vi "EXTI_IO_ISR.vi"(11 "Interrupt_Flag":T1) -> ()   [LabVIEW 2011]
uses:
  D:/National Instruments/LabVIEW 2011/Targets/Keil/Embedded/RealView/Generic/My_ARM_Starter_Board/STM32_DriverVI_Interface/Interrupt/Interrupt_ISR.ctl
  <vilib>/eio/EIO_TerminalDirection.ctl
  <vilib>/STM32_DriverVI_Interface_F4/Interrupt/Interrupt_Flag_F4.ctl
  <vilib>/STM32_DriverVI_Interface_F4/GPIO_EIO/GPI_EIO_Inner_F4.vi
  <vilib>/STM32_DriverVI_Interface_F4/GPIO_EIO/GPO_EIO_Inner_F4.vi
  <vilib>/eio/EIONode/EIONode.xnode
panel:
  # "说明：\n这是一个标准的中断模板 VI，用户可以直接使用,\n在相应的Case语句里面实现相应的中断服务程序即可！\n\n双击打开这个VI之后，另存为副本，名称不变，将其保存\n并添加到自己的项目浏览器中，然后在程序生成规范中进行\n属性设置！"
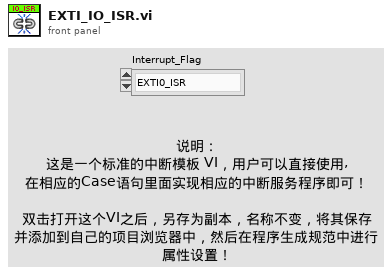
[diagram p1: front panel]
types:
  T1 = typedef "Interrupt_ISR.ctl" = enum8{"EXTI0_ISR", "EXTI1_ISR", "EXTI2_ISR", "EXTI3_ISR", "EXTI4_ISR", "EXTI5_ISR", "EXTI6_ISR", "EXTI7_ISR", "EXTI8_ISR", "EXTI9_ISR", "EXTI10_ISR", "EXTI11_ISR", "EXTI12_ISR", "EXTI13_ISR", "EXTI14_ISR", "EXTI15_ISR"}
  T2 = enum8{"P0", "P1", "P2", "P3", "P4", "P5", "P6", "P7", "P8", "P9", "P10", "P11", "P12", "P13", "P14", "P15"}
  T3 = typedef "Interrupt_Flag_F4.ctl" = enum8{"EXTI0_Flag", "EXTI1_Flag", "EXTI2_Flag", "EXTI3_Flag", "EXTI4_Flag", "EXTI5_Flag", "EXTI6_Flag", "EXTI7_Flag", "EXTI8_Flag", "EXTI9_Flag", "EXTI10_Flag", "EXTI11_Flag", "EXTI12_Flag", "EXTI13_Flag", "EXTI14_Flag", "EXTI15_Flag"}
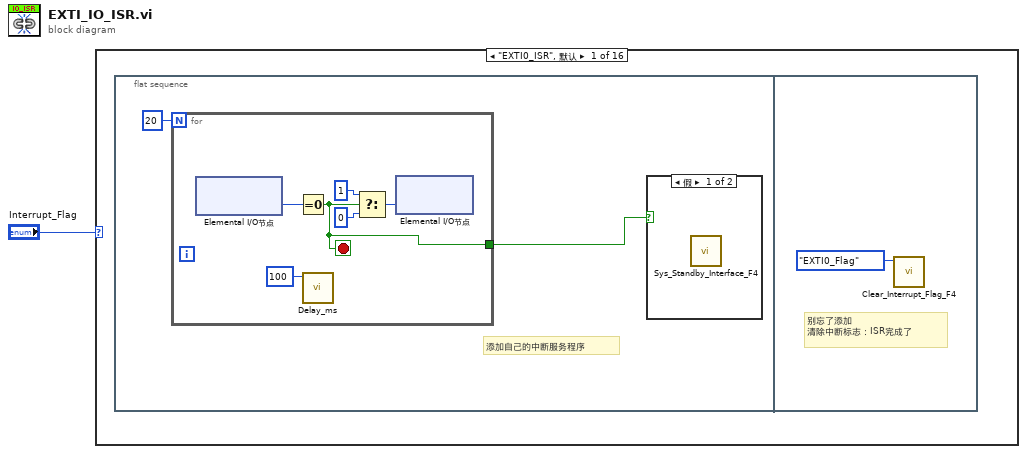
[diagram p0: block diagram]
diagram:
  n1 = case shown="\"EXTI0_ISR\", 默认" "Interrupt_Flag" {
    frame "EXTI0_ISR", Default {
      n2 = flat-sequence {
        frame #0 {
          # "添加自己的中断服务程序"
          n3 = for {
            N: 20 -> [_]
            tunnel: [w6] -> w2
            stop <- w6 stop-if-true
            n4 = xnode "Elemental I/O节点"() -> ("KEY_UP"=w5:u8)  [unwired: 1 in, 1 out]
            n5 = Equal To 0?(x=w5) -> (x = 0?=w6:bool)
            n6 = call <vilib>:"Delay_ms.vi"("time_ms"=u16 100) -> ()  [unwired: 10 in, 1 out]
            n7 = Select(t=u16 1, s=w6, f=u16 0) -> (s? t:f=w7:u16)
            n8 = xnode "Elemental I/O节点"("LED_2"=w7) -> ()  [unwired: 1 in, 1 out]
          }
          n9 = case shown="假" w2 {
            frame False {
              n10 = call <vilib>:"Sys_Standby_Interface_F4.vi"() -> ()  [unwired: 11 in, 1 out]
            }
            frame True {
            }
          }
        }
        frame #1 {
          # "别忘了添加\n清除中断标志：ISR完成了"
          n11 = call <vilib>:"Clear_Interrupt_Flag_F4.vi"("中断标志位"=Interrupt_Flag_F4."EXTI0_Flag") -> ()  [unwired: 10 in, 1 out]
        }
      }
    }
    frame "EXTI1_ISR" {
    }
    frame "EXTI2_ISR" {
    }
    frame "EXTI3_ISR" {
    }
    frame "EXTI4_ISR" {
    }
    frame "EXTI5_ISR" {
    }
    frame "EXTI6_ISR" {
    }
    frame "EXTI7_ISR" {
    }
    frame "EXTI8_ISR" {
    }
    frame "EXTI9_ISR" {
    }
    frame "EXTI10_ISR" {
    }
    frame "EXTI11_ISR" {
    }
    frame "EXTI12_ISR" {
    }
    frame "EXTI13_ISR" {
    }
    frame "EXTI14_ISR" {
    }
    frame "EXTI15_ISR" {
    }
  }
